vi "_WriteSubData_TDMS_SC_CPU.vi"(8 "error in (no error)":errorcluster, 10 "Sub Data in":T1 {"Control"."motor_ctrl_array"."sensor" format="%#.2f"; "Control"."motor_ctrl_array"."setpoint" format="%#.2f"; "Control"."dac_outputs" format="%#.2f"; "PWR"."motor_array"."motor_name" items=["Motor1", "Motor2", "Motor3", "Motor4", "Motor5", "Motor6"]}, 11 "Refnum in":refnum<k34>) -> (0 "error out":errorcluster, 3 "Refnum out":refnum<k34>)   [LabVIEW 2018]
uses:
  TypeDefsSubsea/Sub Data.ctl
  TypeDefsSubsea/Sub Status.ctl
  Shared/Type Defs/ROV States.ctl
  Shared/Type Defs/SMP.ctl
  Shared/Type Defs/PWR.ctl
  Shared/Type Defs/Motor.ctl
  Shared/Type Defs/MotorNames.ctl
  Shared/Type Defs/SmartCard.ctl
  Shared/Type Defs/Box Names.ctl
  TypeDefsSubsea/Sub Control.ctl
  TypeDefsSubsea/Modos Control.ctl
  TypeDefsSubsea/ROV Outputs.ctl
  TypeDefsSubsea/Motor Control.ctl
  TypeDefsSubsea/Type Defs Subsea.lvlib
  TypeDefsTopside/Type Defs Topside.lvlib
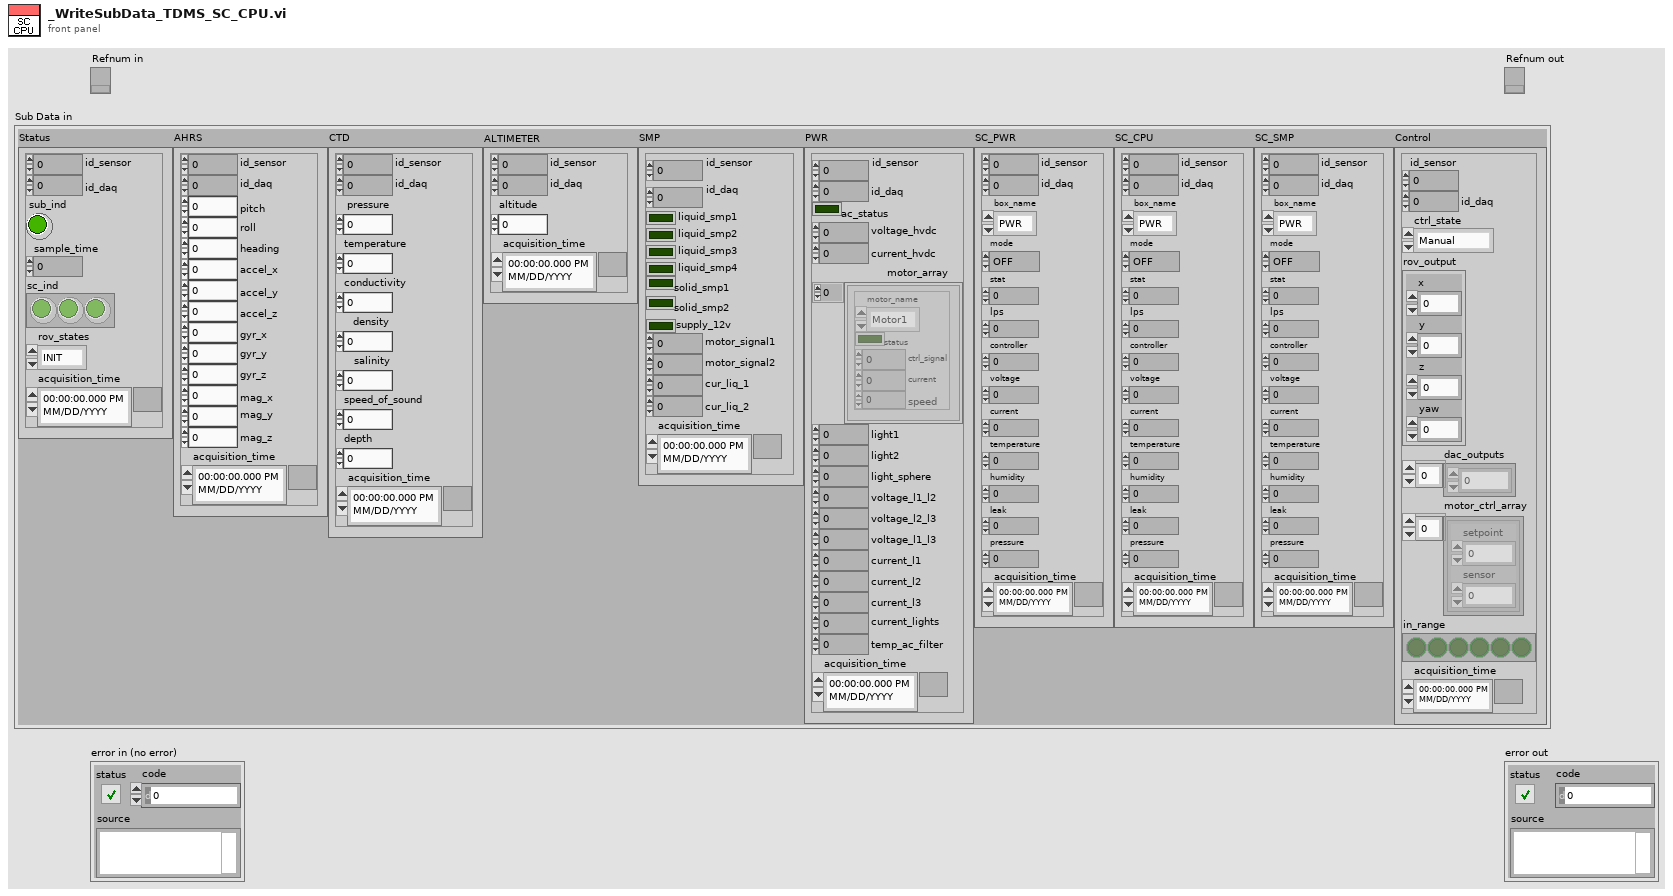
[diagram p1: front panel]
types:
  T1 = typedef "Type Defs Subsea.lvlib/Sub Data.ctl" = cluster{"Status":T2, "AHRS":cluster{"id_sensor":u32, "id_daq":u64, "pitch":dbl, "roll":dbl, "heading":dbl, "accel_x":dbl, "accel_y":dbl, "accel_z":dbl, "gyr_x":dbl, "gyr_y":dbl, "gyr_z":dbl, "mag_x":dbl, "mag_y":dbl, "mag_z":dbl, "acquisition_time":timestamp}, "CTD":cluster{"id_sensor":u32, "id_daq":u64, "pressure":dbl, "temperature":dbl, "conductivity":dbl, "density":dbl, "salinity":dbl, "speed_of_sound":dbl, "depth":dbl, "acquisition_time":timestamp}, "ALTIMETER":cluster{"id_sensor":u32, "id_daq":u64, "altitude":dbl, "acquisition_time":timestamp}, "SMP":T4, "PWR":T5, "SC_PWR":T8, "SC_CPU":T8, "SC_SMP":T8, "Control":T10}
  T2 = typedef "Type Defs Subsea.lvlib/Sub Status.ctl" = cluster{"id_sensor":u32, "id_daq":u32, "sub_ind":bool, "sample_time":i64, "sc_ind":bool[], "rov_states":T3, "acquisition_time":timestamp}
  T3 = typedef "Type Defs Subsea.lvlib/ROV States.ctl" = enum16{"INIT", "IDLE", "TEST", "RUN", "EMERGENCY", "EXIT"}
  T4 = typedef "Type Defs Subsea.lvlib/SMP.ctl" = cluster{"id_sensor":u32, "id_daq":u64, "liquid_smp1":bool, "liquid_smp2":bool, "liquid_smp3":bool, "liquid_smp4":bool, "solid_smp1":bool, "solid_smp2":bool, "supply_12v":bool, "motor_signal1":dbl, "motor_signal2":dbl, "cur_liq_1":dbl, "cur_liq_2":dbl, "acquisition_time":timestamp}
  T5 = typedef "Type Defs Topside.lvlib/PWR.ctl" = cluster{"id_sensor":u32, "id_daq":u64, "ac_status":bool, "voltage_hvdc":dbl, "current_hvdc":dbl, "motor_array":T6[], "light1":dbl, "light2":dbl, "light_sphere":dbl, "voltage_l1_l2":dbl, "voltage_l2_l3":dbl, "voltage_l1_l3":dbl, "current_l1":dbl, "current_l2":dbl, "current_l3":dbl, "current_lights":dbl, "temp_ac_filter":dbl, "acquisition_time":timestamp}
  T6 = typedef "Type Defs Subsea.lvlib/Motor.ctl" = cluster{"motor_name":T7, "status":bool, "ctrl_signal":dbl, "current":dbl, "speed":dbl}
  T7 = typedef "Type Defs Subsea.lvlib/MotorNames.ctl" = u16
  T8 = typedef "Type Defs Subsea.lvlib/SmartCard.ctl" = cluster{"id_sensor":u32, "id_daq":u64, "box_name":T9, "mode":enum16{"OFF", "STANDBY", "TESTING", "RUN", "EMERGENCY"}, "stat":dbl, "lps":dbl, "controller":dbl, "voltage":dbl, "current":dbl, "temperature":dbl, "humidity":dbl, "leak":dbl, "pressure":dbl, "acquisition_time":timestamp}
  T9 = typedef "Type Defs Subsea.lvlib/Box Names.ctl" = enum16{"PWR", "CPU", "SMP"}
  T10 = typedef "Type Defs Subsea.lvlib/Sub Control.ctl" = cluster{"id_sensor":u32, "id_daq":u64, "ctrl_state":T11, "rov_output":T12, "dac_outputs":dbl[], "motor_ctrl_array":T13[], "in_range":bool[], "acquisition_time":timestamp}
  T11 = typedef "Type Defs Subsea.lvlib/Modos Control.ctl" = enum16{"Manual", "Profundidad", "Altitud", "Rumbo", "P+R"}
  T12 = typedef "Type Defs Subsea.lvlib/ROV Outputs.ctl" = cluster{"x":dbl, "y":dbl, "z":dbl, "yaw":dbl}
  T13 = typedef "Type Defs Subsea.lvlib/Motor Control.ctl" = cluster{"setpoint":dbl, "sensor":dbl}
  T14 = enum16{"OFF", "STANDBY", "TESTING", "RUN", "EMERGENCY"}
  T15 = enum16{"OFF", "STANDBY", "TESTING", "RUN", "EMERGENCY"}[]
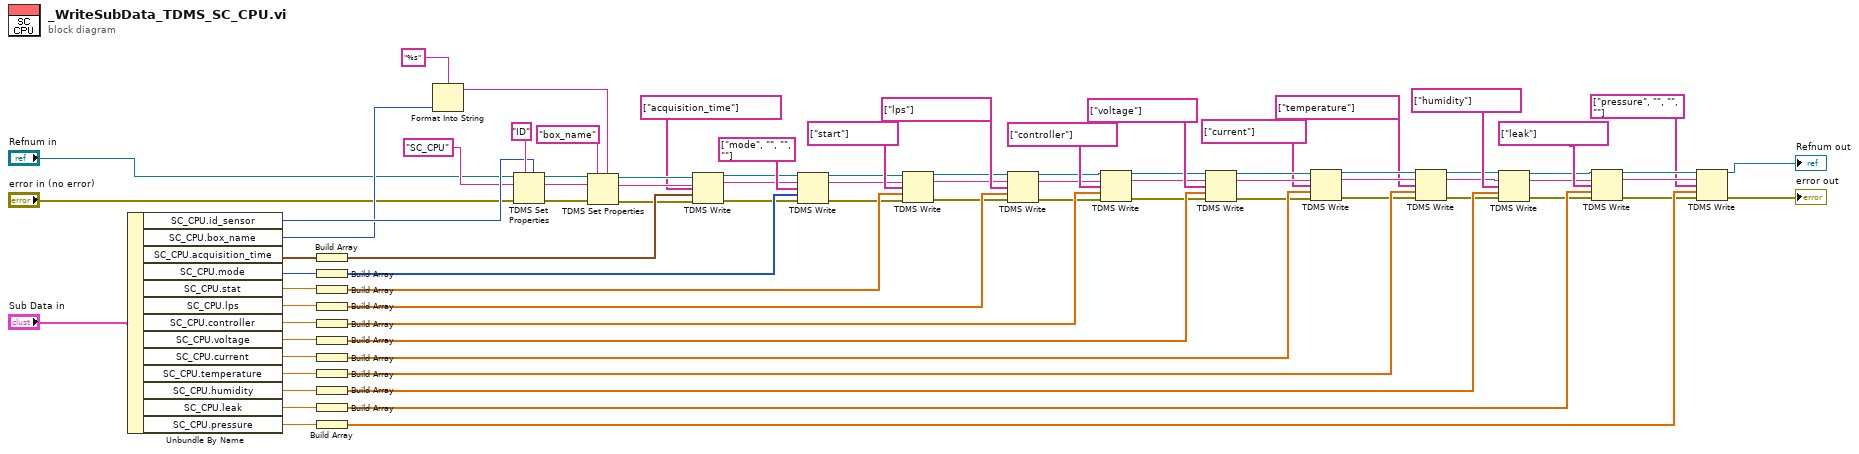
[diagram p0: block diagram]
diagram:
  n1 = Unbundle By Name("Sub Data in") -> ("SC_CPU.id_sensor"=w21:u32, "SC_CPU.box_name"=w15:T9, "SC_CPU.acquisition_time"=w69:timestamp, "SC_CPU.mode"=w70:T14, "SC_CPU.stat"=w9:dbl, "SC_CPU.lps"=w8:dbl, "SC_CPU.controller"=w7:dbl, "SC_CPU.voltage"=w6:dbl, "SC_CPU.current"=w5:dbl, "SC_CPU.temperature"=w4:dbl, "SC_CPU.humidity"=w3:dbl, "SC_CPU.leak"=w2:dbl, "SC_CPU.pressure"=w1:dbl)
  n2 = Build Array(w69) -> (w71:timestamp[])
  n3 = Build Array(w70) -> (w72:T15)
  n4 = Build Array(w9) -> (w73:dbl[])
  n5 = Build Array(w8) -> (w74:dbl[])
  n6 = Build Array(w7) -> (w75:dbl[])
  n7 = Build Array(w6) -> (w76:dbl[])
  n8 = Build Array(w5) -> (w77:dbl[])
  n9 = Build Array(w4) -> (w78:dbl[])
  n10 = Build Array(w3) -> (w79:dbl[])
  n11 = Build Array(w2) -> (w80:dbl[])
  n12 = Build Array(w1) -> (w81:dbl[])
  n13 = Format Into String(format string="%s", w15) -> (resulting string=w16:string)  [unwired: 2 in, 1 out]
  n14 = TDMS Set Properties(5:w21, 7:"ID", 8:"error in (no error)", 10:"SC_CPU" ("group name in (Untitled)"), 11:"Refnum in") -> (0:w24:errorcluster, 2:w19:string, 3:w23:refnum<k34>)  [unwired: 1 in, 1 out]
  n15 = TDMS Set Properties(5:w16, 7:"box_name", 8:w24, 10:w19, 11:w23) -> (0:w32:errorcluster, 2:w31:string, 3:w30:refnum<k34>)  [unwired: 1 in, 1 out]
  n16 = TDMS Write(0:w30, 5:w31, 7:string[] ["acquisition_time"] ("channel name(s) in (Untitled)"), 9:w71, 11:w32) -> (4:w26:refnum<k34>, 6:w25:string, 15:w27:errorcluster)  [unwired: 1 in, 1 out]
  n17 = TDMS Write(0:w26, 5:w25, 7:string[] ["mode", "", "", ""] ("channel name(s) in (Untitled)"), 9:w72, 11:w27) -> (4:w37:refnum<k34>, 6:w36:string, 15:w38:errorcluster)  [unwired: 1 in, 1 out]
  n18 = TDMS Write(0:w37, 5:w36, 7:string[] ["start"] ("channel name(s) in (Untitled)"), 9:w73, 11:w38) -> (4:w34:refnum<k34>, 6:w33:string, 15:w35:errorcluster)  [unwired: 1 in, 1 out]
  n19 = TDMS Write(0:w34, 5:w33, 7:string[] ["lps"] ("channel name(s) in (Untitled)"), 9:w74, 11:w35) -> (4:w52:refnum<k34>, 6:w53:string, 15:w67:errorcluster)  [unwired: 1 in, 1 out]
  n20 = TDMS Write(0:w52, 5:w53, 7:string[] ["controller"] ("channel name(s) in (Untitled)"), 9:w75, 11:w67) -> (4:w50:refnum<k34>, 6:w51:string, 15:w49:errorcluster)  [unwired: 1 in, 1 out]
  n21 = TDMS Write(0:w50, 5:w51, 7:string[] ["voltage"] ("channel name(s) in (Untitled)"), 9:w76, 11:w49) -> (4:w44:refnum<k34>, 6:w45:string, 15:w43:errorcluster)  [unwired: 1 in, 1 out]
  n22 = TDMS Write(0:w44, 5:w45, 7:string[] ["current"] ("channel name(s) in (Untitled)"), 9:w77, 11:w43) -> (4:w47:refnum<k34>, 6:w48:string, 15:w46:errorcluster)  [unwired: 1 in, 1 out]
  n23 = TDMS Write(0:w47, 5:w48, 7:string[] ["temperature"] ("channel name(s) in (Untitled)"), 9:w78, 11:w46) -> (4:w62:refnum<k34>, 6:w64:string, 15:w63:errorcluster)  [unwired: 1 in, 1 out]
  n24 = TDMS Write(0:w62, 5:w64, 7:string[] ["humidity"] ("channel name(s) in (Untitled)"), 9:w79, 11:w63) -> (4:w59:refnum<k34>, 6:w60:string, 15:w65:errorcluster)  [unwired: 1 in, 1 out]
  n25 = TDMS Write(0:w59, 5:w60, 7:string[] ["leak"] ("channel name(s) in (Untitled)"), 9:w80, 11:w65) -> (4:w57:refnum<k34>, 6:w58:string, 15:w56:errorcluster)  [unwired: 1 in, 1 out]
  n26 = TDMS Write(0:w57, 5:w58, 7:string[] ["pressure", "", "", ""] ("channel name(s) in (Untitled)"), 9:w81, 11:w56) -> (4:→"Refnum out":refnum<k34>, 15:→"error out":errorcluster)  [unwired: 1 in, 2 out]
